vi "using filters.vi"() -> ()   [LabVIEW 2013]
panel:
  out "Image Out":T1(plugin-control)
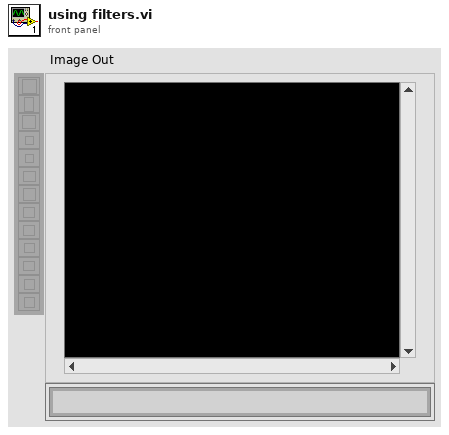
[diagram p1: front panel]
types:
  T1 = typedef "IMAQ Image.ctl" = refnum<image>
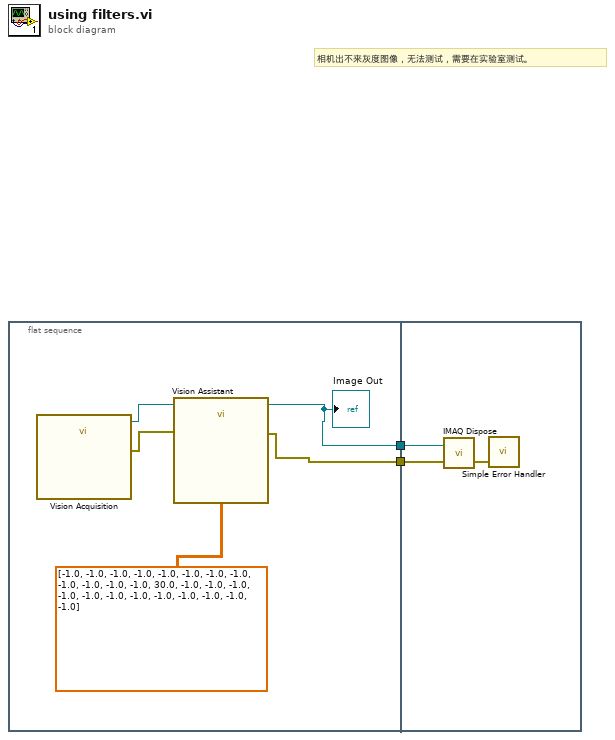
[diagram p0: block diagram]
diagram:
  # "相机出不来灰度图像，无法测试，需要在实验室测试。"
  n1 = flat-sequence {
    tunnel: [w5] -> w2
    tunnel: [w4] -> w1
    tunnel: w2 -> [w8]
    tunnel: w1 -> [w9]
    frame #0 {
      n2 = call "Vision Acquisition"() -> ("Image Out"=w7:T1, "error out"=w6:errorcluster)  [unwired: 26 in]
      n3 = call "Vision Assistant"("Image In"=w7, "Kernel (Filters 2)"=sgl[][] [[-1.0, -1.0, -1.0, -1.0, -1.0], [-1.0, -1.0, -1.0, -1.0, -1.0], [-1.0, -1.0, 30.0, -1.0, -1.0], [-1.0, -1.0, -1.0, -1.0, -1.0], [-1.0, -1.0, -1.0, -1.0, -1.0]], "error in"=w6) -> ("Image Out"=w4:T1, "error out"=w5:errorcluster)  [unwired: 23 in]
      "Image Out" <- w4
    }
    frame #1 {
      n4 = call "IMAQ Dispose"("Image"=w9, "error in (no error)"=w8) -> ("error out"=w10:errorcluster)  [unwired: 4 in]
      n5 = call <vilib>:"Simple Error Handler.vi"("error in (no error)"=w10) -> ()  [unwired: 4 in, 5 out]
    }
  }
